vi "Resolve-message-type.vi"(8 "error in (no error)":errorcluster, 11 "Message":refnum<class "Message.lvclass">) -> (0 "error out":errorcluster, 2 "Message type":T1, 3 "Message dup":refnum<class "Message.lvclass">)   [LabVIEW 2013, in "Client.lvlib" / "Client.lvclass"]
uses:
  Client.lvclass
  Messages/Sources/Message.lvclass
  Supported-messages.ctl
  Messages/Sources/Message.lvclass/Message.ctl
  Custom-errors.ctl
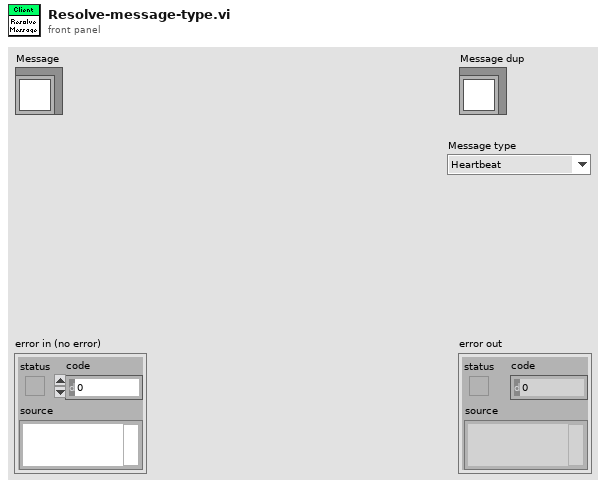
[diagram p1: front panel]
types:
  T1 = typedef "Client.lvlib/Client.lvclass/Supported-messages.ctl" = enum16{"Heartbeat", "Error", "Start client", "Client stopped", "Action", "Query status", "Send status", "Get clients"}
  T2 = typedef "Client.lvlib/Client.lvclass/Custom-errors.ctl" = enum16{"No error", "Command not recognized", "Invalid input", "Timeout", "Not implemented", "Unsupported message", "Unsupported client", "Unsupported action"}
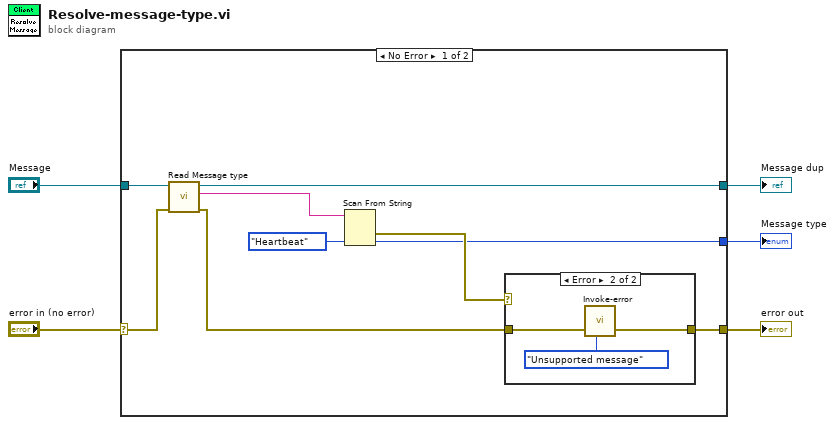
[diagram p0: block diagram]
diagram:
  n1 = case shown="No Error" "error in (no error)" {
    selector: "error in (no error)" -> [w10 w19]
    tunnel: [w7 w19] -> w4
    tunnel: "Message" -> [w14 w18]
    tunnel: [w13 w18] -> w2
    tunnel: [w6 _] -> w1
    frame No Error {
      n2 = call "Read Message type.vi"("error in (no error)"=w10, "Message in"=w14) -> ("error out"=w8:errorcluster, "String"=w11:string, "Message out"=w13:refnum<class "Message.lvclass">)  [unwired: 7 in]
      n3 = Scan From String(input string=w11, default 1=Supported-messages."Heartbeat" ("Type")) -> (error out=w9:errorcluster, output 1=w6:T1)  [unwired: 3 in, 2 out]
      n4 = case shown="Error" w9 {
        tunnel: w8 -> [w15 w17]
        tunnel: [w15 w17] -> w7
        frame No Error {
        }
        frame Error {
          n5 = call "Invoke-error.vi"("Error"=Custom-errors."Unsupported message") -> ()  [unwired: 10 in, 1 out]
        }
      }
    }
    frame Error {
    }
  }
  "error out" <- w4
  "Message dup" <- w2
  "Message type" <- w1
